vi "Lockin.DAQ.Create AI Tasks.vi"(8 "error in (no error)":errorcluster, 11 "Lockin.DAQ":refnum<class "Lockin.DAQ.lvclass">) -> (0 "error out":errorcluster, 3 "Lockin.DAQ":refnum<class "Lockin.DAQ.lvclass">)   [LabVIEW 2019, in "Lockin.DAQ.lvclass"]
uses:
  Lockin.DAQ.lvclass
  Lockin.DAQ.lvclass/Lockin.DAQ.ctl
  <vilib>/DAQmx/create/channels.llb/DAQmx Create Channel (AI-Voltage-Basic).vi
  <resource>/objmgr/daqmx.rc
panel:
  out "Current Size":i32
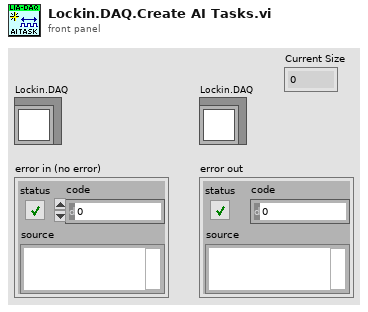
[diagram p1: front panel]
types:
  T1 = typedef "Lockin.DAQ.lvclass/AI.config-array.ctl" = T2[]
  T2 = typedef "Lockin.DAQ.lvclass/AI.config-cluster.ctl" = cluster{"AI.channels":tag, "AI.Coupling":T3, "AI.Range":T4, "input terminal configuration":i32, "DAQ Type":T5}
  T3 = typedef "Lockin.DAQ.lvclass/AI.coupling-enum.ctl" = u16
  T4 = typedef "Lockin.DAQ.lvclass/446xAI-enum.ctl" = enum16{"±0.316", "±1.00", "±3.16", "±10.0", "±31.6", "±42.4"}
  T5 = typedef "Lockin.DAQ.lvclass/DAQType-enum.ctl" = enum16{"None", "USB 4431", "PXI 446x"}
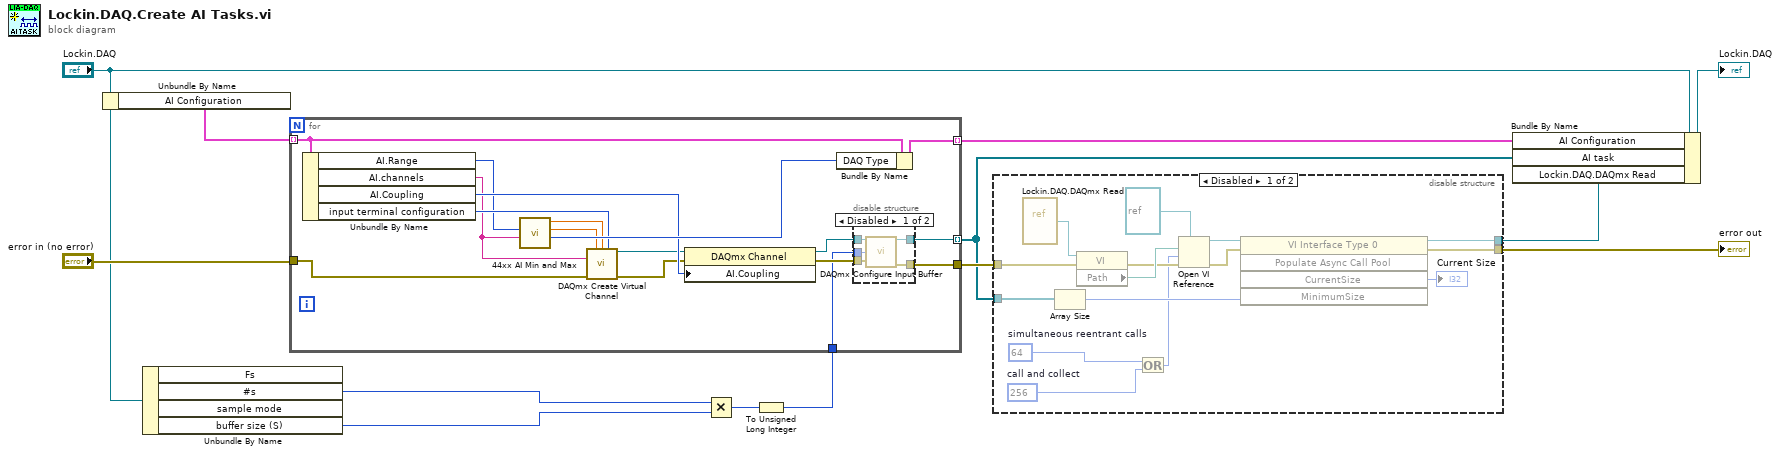
[diagram p0: block diagram]
diagram:
  n1 = Unbundle By Name("Lockin.DAQ") -> ("AI Configuration"=w5:T1)
  n2 = Unbundle By Name("Lockin.DAQ") -> ("#s"=w10:i32, "buffer size (S)"=w9:u32)  [unwired: 2 out]
  n3 = Multiply(x=w10, y=w9) -> (x*y=w11:u32)
  n4 = To Unsigned Long Integer(number=w11) -> (unsigned 32bit integer=w8:u32)
  n5 = for {
    tunnel: [w14] -> w7 mode=indexing
    tunnel: w5 -> [w21] mode=indexing
    tunnel: "error in (no error)" -> [w22]
    tunnel: [w19] -> w4
    tunnel: w8 -> [w17]
    tunnel: [w16] -> w1 mode=indexing
    n6 = Unbundle By Name(w21) -> ("AI.Range"=w27:T4, "AI.channels"=w15:tag, "AI.Coupling"=w28:T3, "input terminal configuration"=w29:i32)
    n7 = call "44xx AI Min and Max.vi"("AI.channels"=w15, "446x AI"=w27) -> ("DAQ Type"=w30:T5, "AI.Max"=w25:dbl, "AI.Min"=w26:dbl)  [unwired: 7 in]
    n8 = call-poly <vilib>:"DAQmx Create Virtual Channel.vi"("maximum value"=w25, "minimum value"=w26, "input terminal configuration"=w29, "physical channels"=w15, "error in"=w22) -> ("task out"=w23:refnum<k21>, "error out"=w24:errorcluster)  [unwired: 9 in]
    n9 = property class="DAQmx Channel"(reference=w23, error in=w24, "AI.Coupling"=w28) -> (reference out=w18:refnum<k21>, error out=w20:errorcluster)
    n10 = Bundle By Name(cluster=w21, "DAQ Type"=w30) -> (w14:T2)
    n11 = disable-structure shown="Disabled" {
      disable-tunnel: w20 -> [w35 w36]
      disable-tunnel: [w34 w36] -> w19
      disable-tunnel: w18 -> [w33 w37]
      disable-tunnel: w17 -> [w32 _]
      disable-tunnel: [w31 w37] -> w16
      frame Disabled {
        n12 = call <vilib>:"DAQmx Configure Input Buffer.vi"("task/channels in"=w33, "buffer size (in samples per channel)"=w32, "error in"=w35) -> ("task out"=w31:refnum<k21>, "error out"=w34:errorcluster)  [unwired: 11 in]
      }
      frame Enabled {
      }
    }
  }
  n13 = disable-structure shown="Disabled" {
    disable-tunnel: w4 -> [w47 w53]
    disable-tunnel: [w46 w53] -> w3
    disable-tunnel: [w45 _] -> w2
    disable-tunnel: w1 -> [w42 _]
    frame Disabled {
      w40 = 64  # simultaneous reentrant calls
      w38 = 256  # call and collect
      n14 = vi-ref "Lockin.DAQ.DAQmx Read.vi"() -> (w43:refnum<vi>)
      n15 = Array Size(array=w42) -> (size(s)=w41:i32)
      n16 = property class="VI"(reference=w43, error in=w47) -> (error out=w51:errorcluster, "Path"=w52:path)  [unwired: 1 out]
      n17 = Or(x=w40, y=w38) -> (x .or. y?=w39:i32)
      n18 = Open VI Reference(type specifier VI Refnum (for type only)=refnum<vi> refnum, vi path=w52, options=w39, error in (no error)=w51) -> (vi reference=w49:refnum<vi>, error out=w48:errorcluster)  [unwired: 2 in]
      n19 = invoke class="VI Interface Type 0" method="Populate Async Call Pool"(reference=w49, error in=w48, "MinimumSize"=w41) -> (reference out=w45:refnum<vi>, error out=w46:errorcluster, "CurrentSize"=→"Current Size":i32)  [unwired: 2 in, 2 out]
    }
    frame Enabled {
    }
  }
  "error out" <- w3
  n20 = Bundle By Name(cluster="Lockin.DAQ", "AI Configuration"=w7, "AI task"=w1, "Lockin.DAQ.DAQmx Read"=w2) -> (→"Lockin.DAQ":refnum<class "Lockin.DAQ.lvclass">)
